vi "Async.Engine.Initialize.vi"(5 "Plugin Name":string, 6 "Timeout (ms) (5000)":u16=5000, 7 "Error Log Settings":T2, 8 "error in":errorcluster, 9 "PluginAPIs":T1=refnum, 10 "Processes":cluster{"VI":refnum<vi>, "Parameters":variant}[](array[cluster]), 11 "Compiled.InlineAsync.Settings":variant) -> (0 "error out":errorcluster, 3 "Async":refnum<class "VS Plugin Inline Async API.lvclass">)   [LabVIEW 2023, in "VS Plugin Inline Async API.lvlib" / "VS Plugin Inline Async API.lvclass"]
uses:
  VS Plugin Inline Async API.lvclass
  VS Plugin Inline Async API.lvclass/VS Plugin Inline Async API.ctl
  Error Handling Process/Display and Log Process.vi
  VS Plugin Inline Async API.lvlib
  _Plugin Data Access Engine/Plugin Data Access Engine/Plugin Data Access Engine.lvclass
  Types/Error Handling Settings.ctl
  <userlib>/PluginCore_v1.lvlibp/iPluginAPIs/iPluginAPIs.lvclass
  _PluginCore/Types/Plugin API.ctl
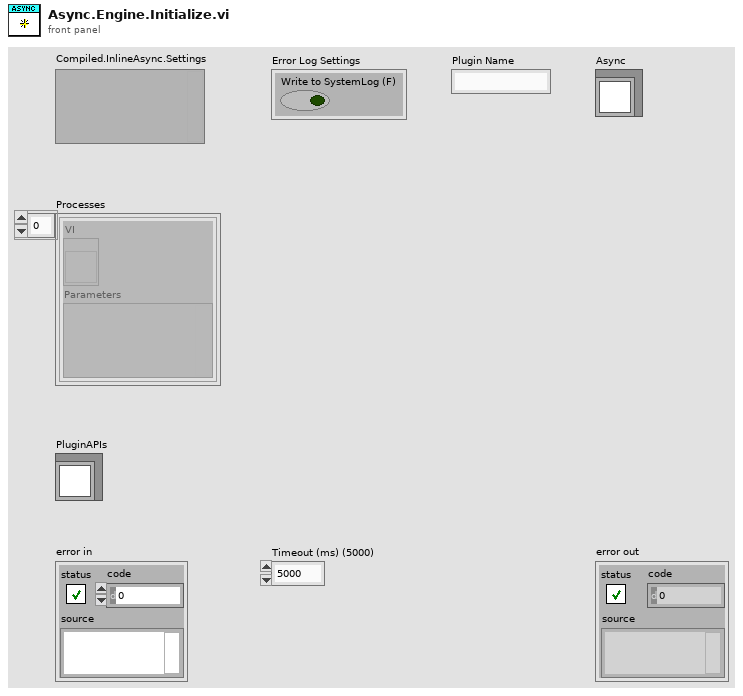
[diagram p1: front panel]
types:
  T1 = typedef "Plugin API.ctl" = refnum<class "iPluginAPIs.lvclass">
  T2 = typedef "VS Plugin Inline Async API.lvlib/VS Plugin Inline Async API.lvclass/Error Handling Settings.ctl" = cluster{"Write to SystemLog (F)":bool}
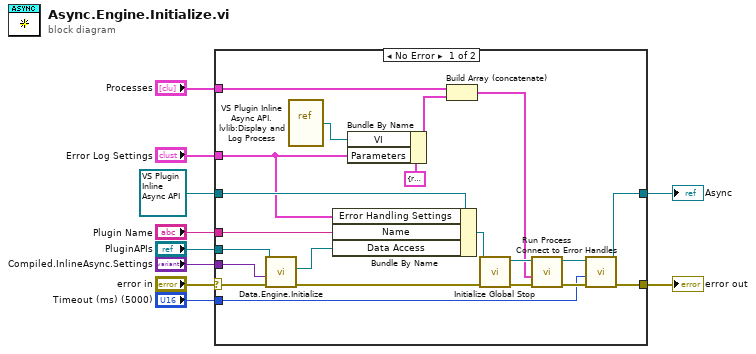
[diagram p0: block diagram]
diagram:
  n1 = case shown="No Error" "error in" {
    selector: "error in" -> [w19 w33]
    tunnel: [w28 w33] -> w9
    tunnel: [w26 w32] -> w3
    tunnel: refnum<class "VS Plugin Inline Async API.lvclass"> refnum ("Async in") -> [w31 w32]
    tunnel: "Processes" -> [w30 _]
    tunnel: "Error Log Settings" -> [w17 _]
    tunnel: "Timeout (ms) (5000)" -> [w16 _]
    tunnel: "PluginAPIs" -> [w15 _]
    tunnel: "Compiled.InlineAsync.Settings" -> [w13 _]
    tunnel: "Plugin Name" -> [w12 _]
    frame No Error {
      n2 = call "Data.Engine.Initialize.vi"("error in"=w19, "Compiled.InlineAsync.Settings"=w13, "PluginAPIs"=w15) -> ("error out"=w14:errorcluster, "Data Access Engine"=w11:refnum<class "Plugin Data Access Engine.lvclass">)  [unwired: 7 in]
      n3 = vi-ref "VS Plugin Inline Async API.lvlib:Display and Log Process.vi"() -> (w24:refnum<vi>)
      n4 = Bundle By Name(cluster=w31, "Error Handling Settings"=w17, "Name"=w12, "Data Access"=w11) -> (w18:refnum<class "VS Plugin Inline Async API.lvclass">)
      n5 = Bundle By Name(cluster=cluster{"VI":refnum<vi>, "Parameters":variant} {"VI"=refnum, "Parameters"=variant} ("Process"), "VI"=w24, "Parameters"=w17) -> (w23:cluster{"VI":refnum<vi>, "Parameters":variant})
      n6 = Build Array (concatenate)(w30, w23) -> (w20:cluster{"VI":refnum<vi>, "Parameters":variant}[])
      n7 = call "Initialize Global Stop.vi"("error in"=w14, "Async in"=w18) -> ("error out"=w22:errorcluster, "Async out"=w21:refnum<class "VS Plugin Inline Async API.lvclass">)  [unwired: 8 in]
      n8 = call "Run Process.vi"("error in"=w22, "Processes"=w20, "Async in"=w21) -> ("error out"=w29:errorcluster, "Async out"=w27:refnum<class "VS Plugin Inline Async API.lvclass">)  [unwired: 7 in]
      n9 = call "Connect to Error Handles.vi"("error in"=w29, "Timeout (ms)"=w16, "Async in"=w27) -> ("error out"=w28:errorcluster, "Async out"=w26:refnum<class "VS Plugin Inline Async API.lvclass">)  [unwired: 7 in]
    }
    frame Error {
    }
  }
  "error out" <- w9
  "Async" <- w3
